vi "Main_Host.vi"() -> ()   [LabVIEW 2020]
doc: "JSMA Project Wizard 0.2.0.11\nRob Humfeld - JET Engineering\nCopyright (c) 2020, JET Engineering"
uses:
  Main_Host_Status STYP.ctl
  <userlib>/JET Engineering/JET_QSM/Code/Private/JET_QSM - Add State [String API].vi
  <userlib>/JET Engineering/JSMA/Libraries/jMasterTable_Message/jMasterTable_Message - Reset.vi
  <userlib>/JET Engineering/JSMA/Libraries/jMasterTable_Module/jMasterTable_Module - Reset.vi
  <userlib>/JET Engineering/JSMA/Libraries/jMasterTable_Message/jMasterTable_Message - Get-Create Queue.vi
  <userlib>/JET Engineering/JSMA/Libraries/jMasterTable_Subscription/jMasterTable_Subscription - Reset.vi
  <userlib>/JET Engineering/JSMA/Libraries/jMasterTable_Module/jMasterTable_Module - Get-Create Queue.vi
  <userlib>/JET Engineering/JSMA/Libraries/jMasterTable_Module/jMasterTable_Module - Get Table Name.vi
  <vilib>/Utility/error.llb/Trim Whitespace.vi
  <userlib>/JET Engineering/JSMA/Libraries/jMasterShutdownFlag/jFlag_MasterShutdown - Reset.vi
  <vilib>/Utility/error.llb/Error Cluster From Error Code.vi
  Shared/Globals/Main_Host Config GBL.vi
  <userlib>/JET Engineering/JSMA/Libraries/jSubscription Class/jSubscription.lvclass
  <userlib>/JET Engineering/JSMA Exception Handler UI/Module_JSMA_UI_ExceptionHandler.lvclass
  <userlib>/JET Engineering/JSMA/Libraries/jApplication/jApplication.lvclass
  Module_UI_TopLevel/Module_UI_TopLevel.lvclass
panel:
  in  "Status":T1
  out "error out":errorcluster
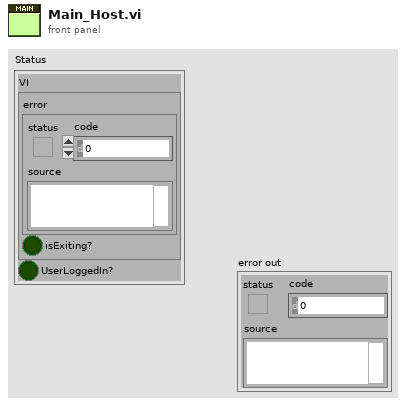
[diagram p1: front panel]
types:
  T1 = typedef "Main_Host_Status STYP.ctl" = cluster{"VI":cluster{"error":errorcluster, "isExiting?":bool}, "UserLoggedIn?":bool}
  T2 = typedef "JET_QSM_Refnum STYP.ctl" = cluster{"state":cluster{"queue":refnum<queue>, "idle":string, "error":string, "STOP":string}, "debug":cluster{"enabled?":bool, "queue":refnum<queue>}, "Invalid.option":T3, "QSM.Name":string}
  T3 = typedef "JET_QSM_InvalidOption STYP.ctl" = enum16{"Ignore", "Dialog", "Error"}
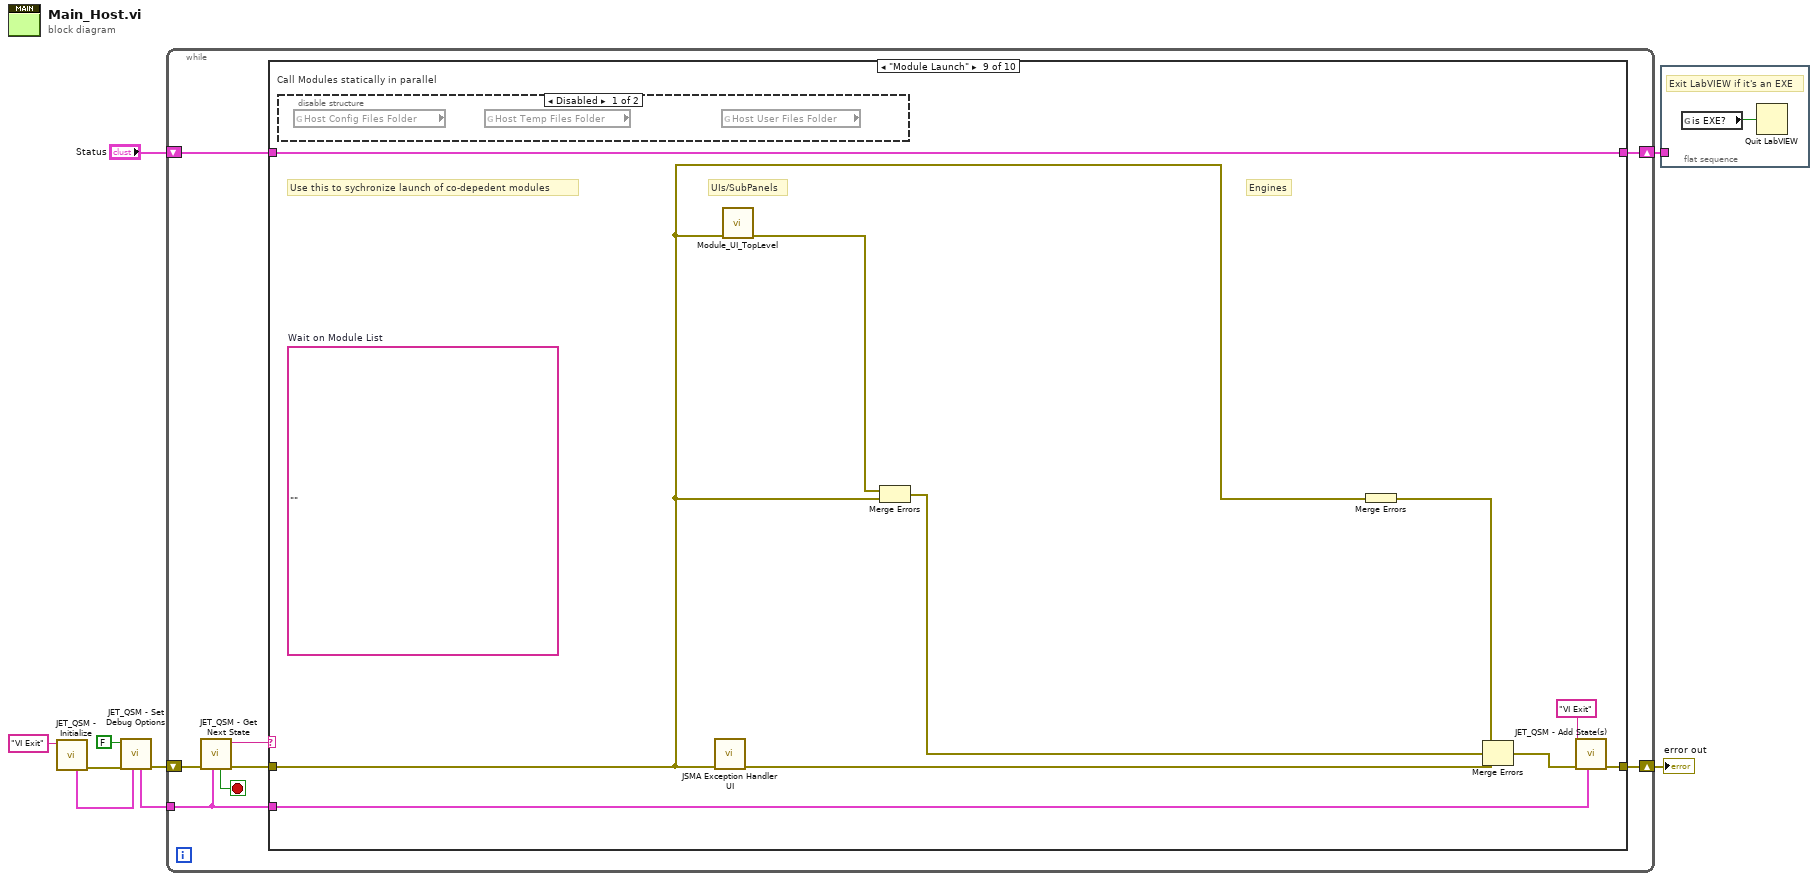
[diagram p0: block diagram]
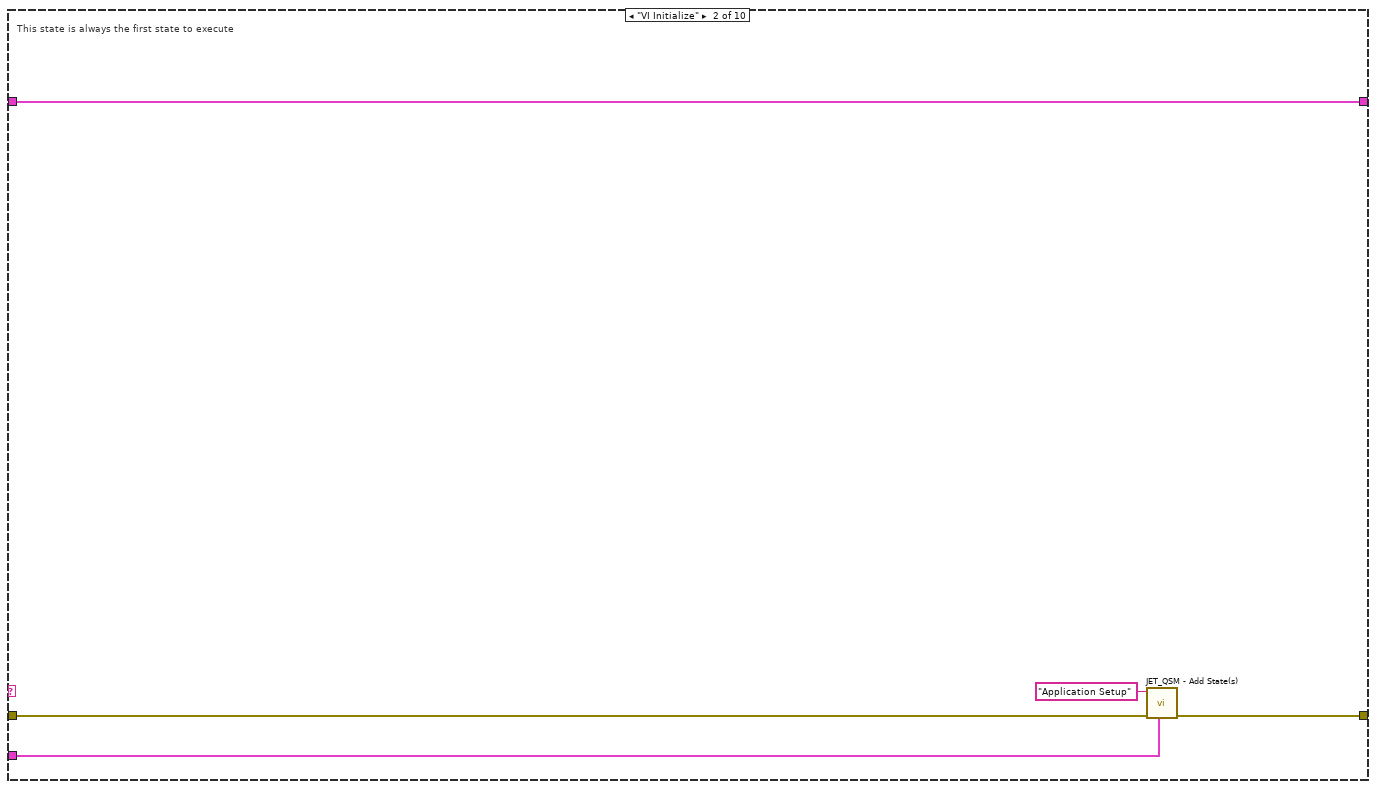
[diagram p3: hidden frame]
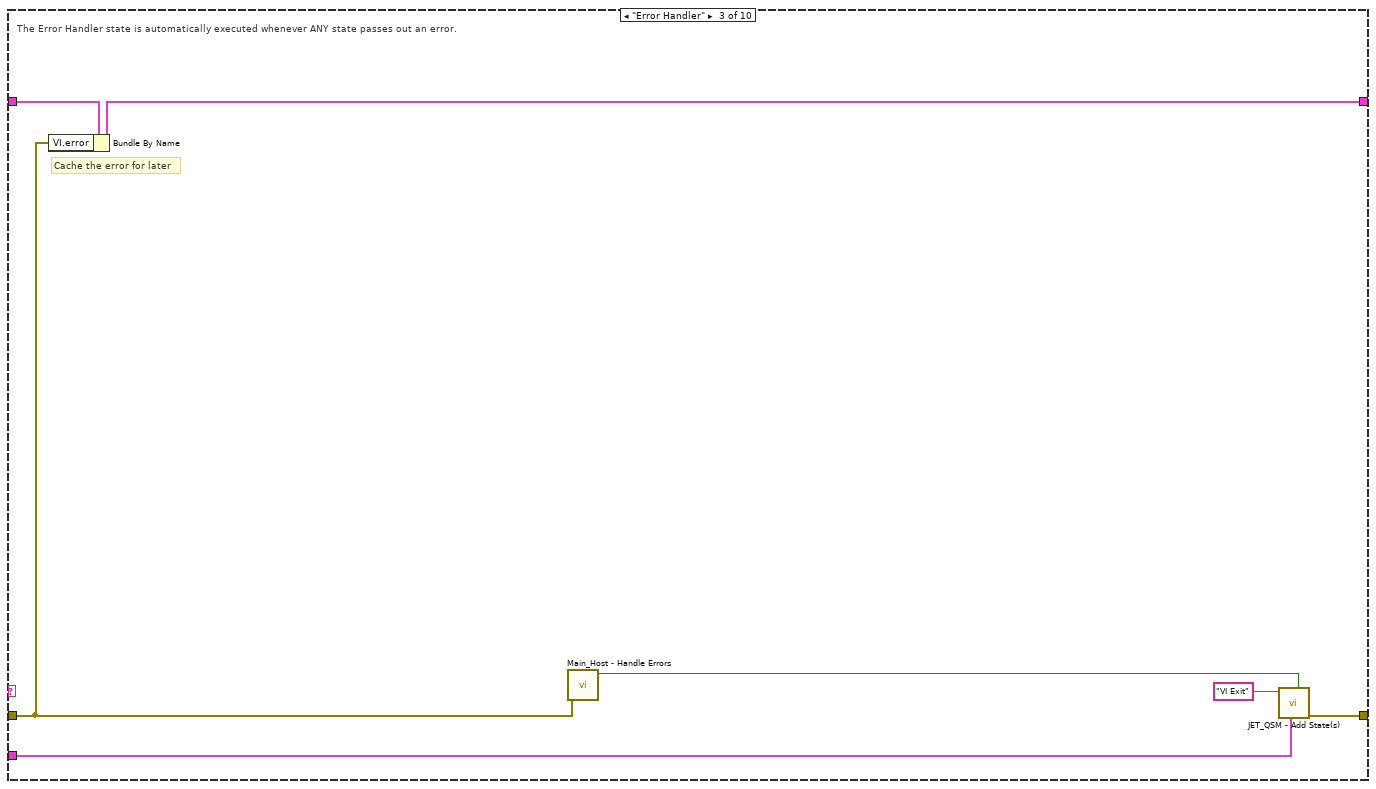
[diagram p4: hidden frame]
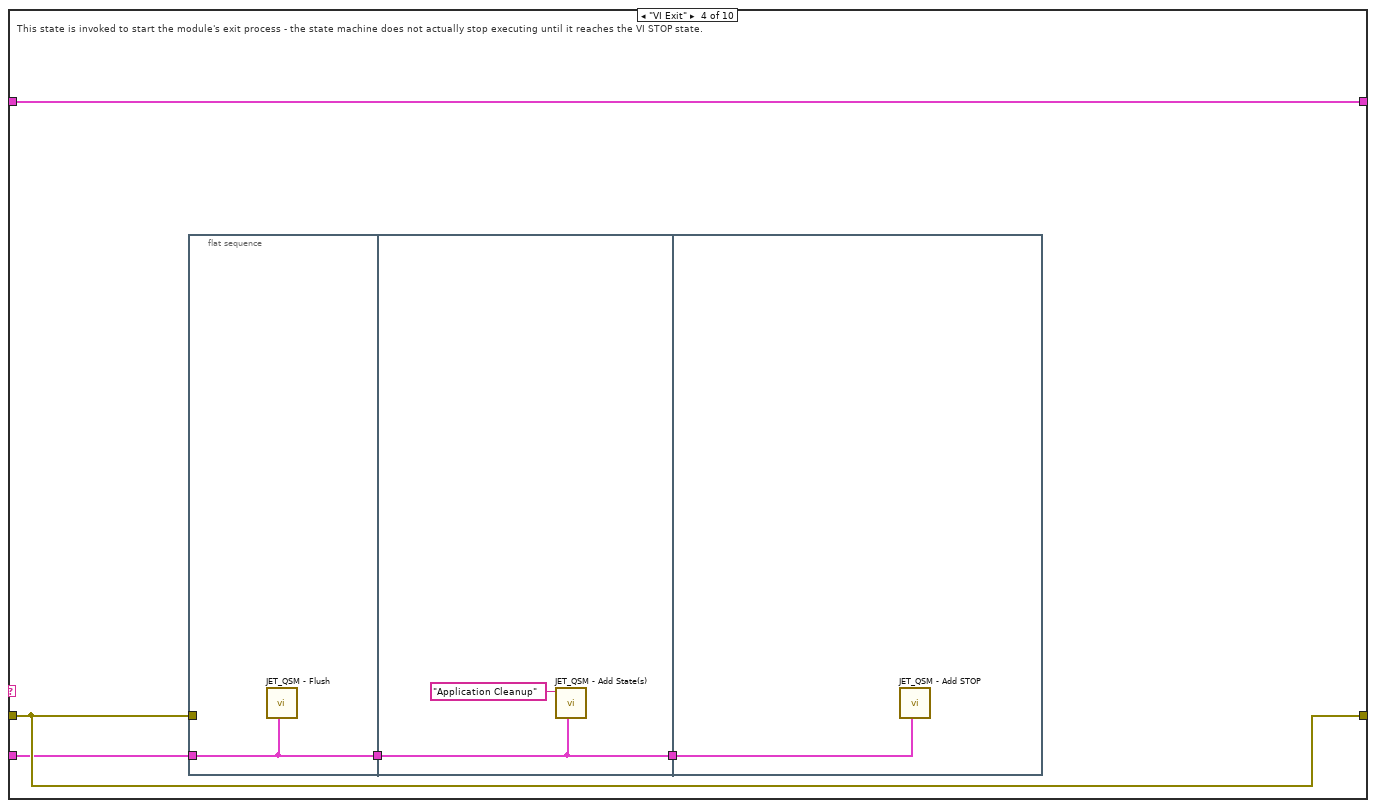
[diagram p5: hidden frame]
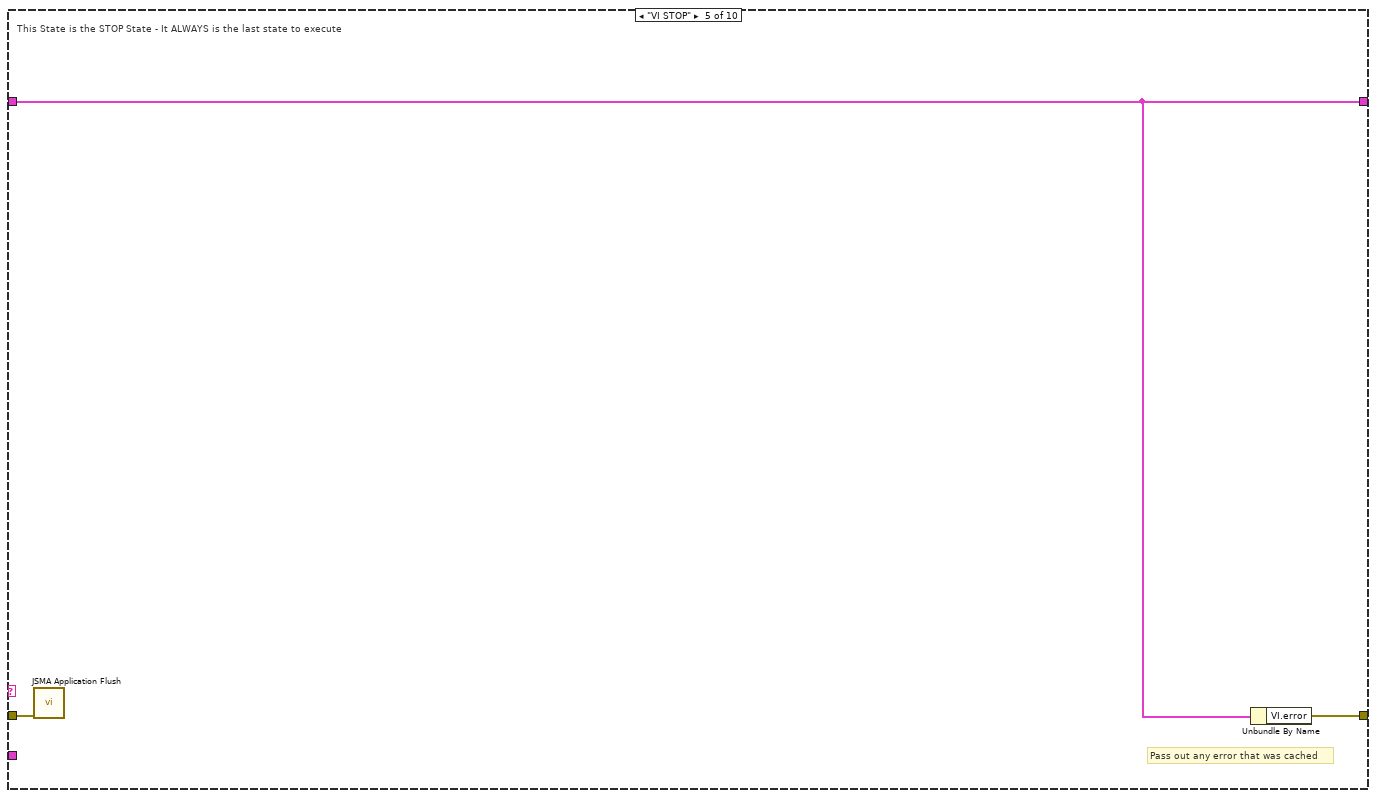
[diagram p6: hidden frame]
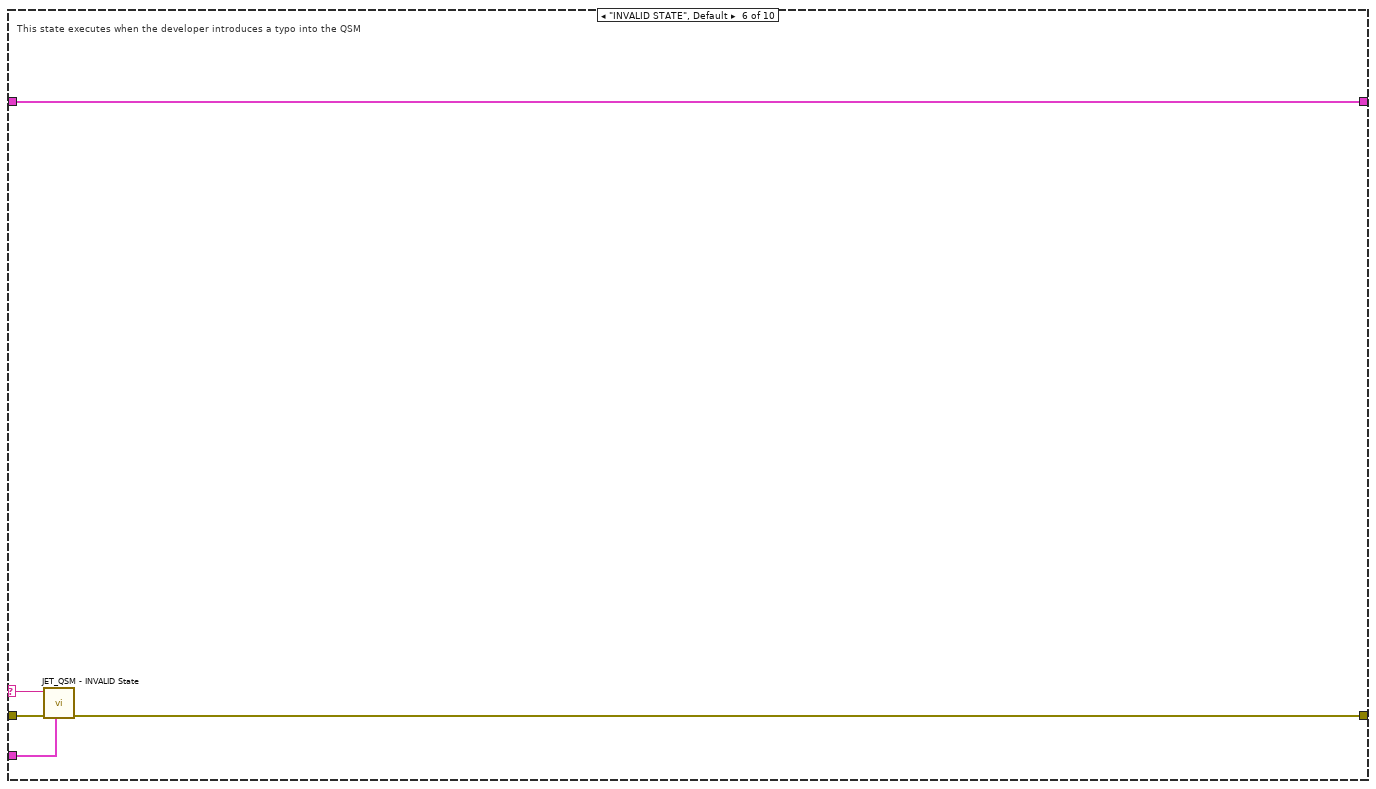
[diagram p7: hidden frame]
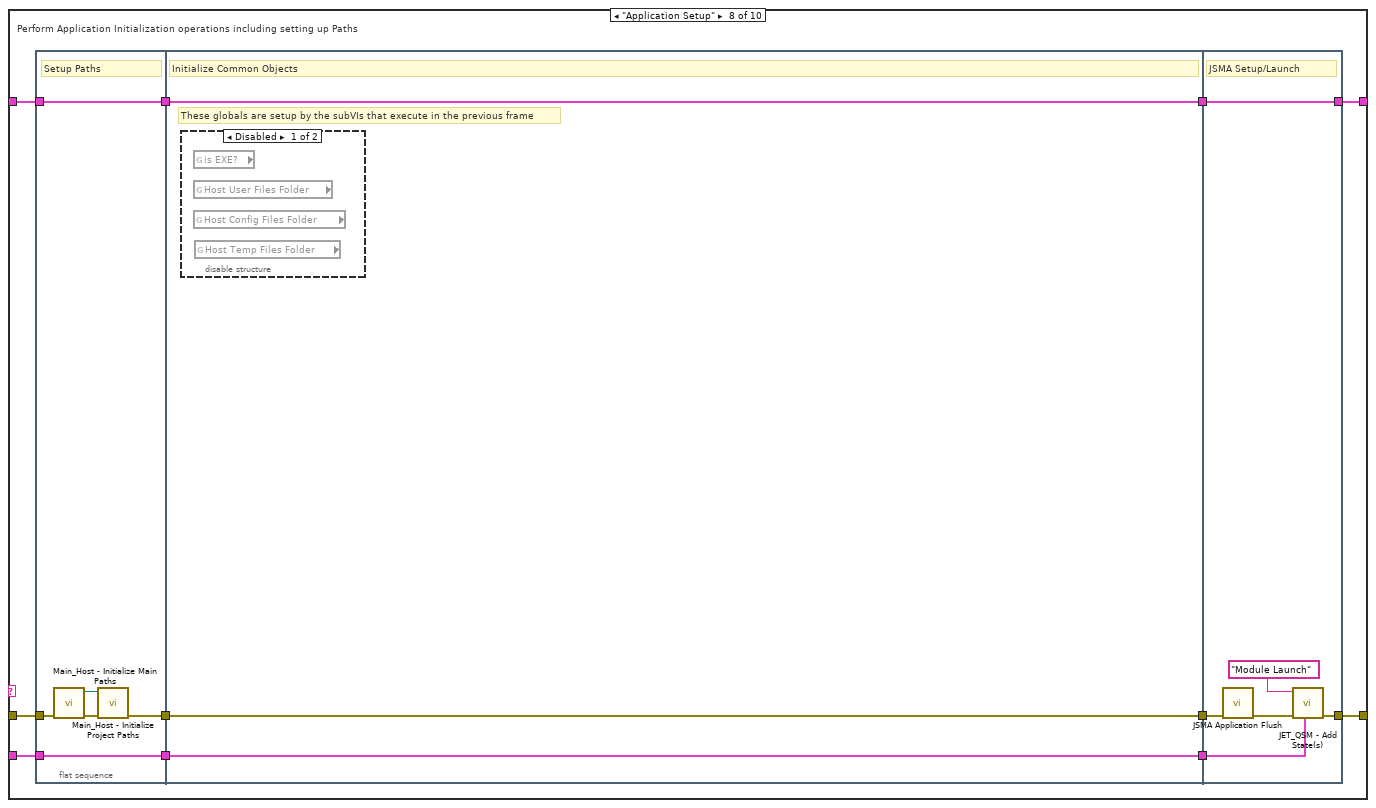
[diagram p9: hidden frame]
diagram:
  n1 = call <userlib>:"JET_QSM - Initialize.vi"("idle state (\"Event Check\")"="VI Exit" ("idle state (\"Event Check\")")) -> ("error out"=w3:errorcluster, "Jet_QSM refnum"=w6:T2)  [unwired: 9 in]
  n2 = call <userlib>:"JET_QSM - Set Debug Options.vi"("Jet_QSM refnum"=w6, "error in (no error)"=w3, "debug.enabled? (F)"=FALSE) -> ("error out"=w4:errorcluster, "Jet_QSM ref"=w5:T2)  [unwired: 7 in]
  n3 = while {
    tunnel: w5 -> [w13]
    shift-right: [w11] -> w2
    shift-left: "Status" -> [w12]
    shift-right: [w10] -> w9
    shift-left: w4 -> [w17]
    stop <- w14 stop-if-true
    n4 = call <userlib>:"JET_QSM - Get Next State.vi"("Jet_QSM refnum"=w13, "error in (no error)"=w17) -> ("error out"=w16:errorcluster, "state"=w15:string, "Stop Loop?"=w14:bool)  [unwired: 5 in, 2 out]
    n5 = case shown="\"Module Launch\"" w15 {
      selector: w15 -> [_ _ _ _ _ w46 _ _ _ _]
      tunnel: w16 -> [w18 w22 w26 w36 w41 w47 w49 w61 w78 w87]
      tunnel: w13 -> [_ w23 w30 w35 _ w45 _ w56 w85 _]
      tunnel: w12 -> [w19 w24 w28 w34 w42 w48 w50 w53 w86 w88]
      tunnel: [w19 w24 w27 w34 w42 w48 w50 w51 w86 w88] -> w11
      tunnel: [w18 w21 w31 w36 w43 w44 w49 w55 w84 w87] -> w10
      frame "------ Standard States ------" {
        # "Standard States are required states for a JET_QSM State Machine\n\nTheir names may be changed; use the Initialize function to specify the new names"
        # "This is a section header; the state is never expected to execute"
      }
      frame "VI Initialize" {
        # "This state is always the first state to execute"
        n6 = call-poly <userlib>:"JET_QSM - Add State(s).vi"("Jet_QSM refnum"=w23, "error in (no error)"=w22, "state(s)"="Application Setup") -> ("error out"=w21:errorcluster)  [unwired: 8 in]
      }
      frame "Error Handler" {
        # "Cache the error for later"
        # "The Error Handler state is automatically executed whenever ANY state passes out an error."
        n7 = Bundle By Name(cluster=w28, "VI.error"=w26) -> (w27:T1)
        n8 = call "Main_Host - Handle Errors.vi"("error in (no error)"=w26) -> ("VI Exit?"=w25:bool)  [unwired: 10 in]
        n9 = call-poly <userlib>:"JET_QSM - Add State(s).vi"("act? (T)"=w25, "Jet_QSM refnum"=w30, "state(s)"="VI Exit") -> ("error out"=w31:errorcluster)  [unwired: 8 in]
      }
      frame "VI Exit" {
        # "This state is invoked to start the module's exit process - the state machine does not actually stop executing until it reaches the VI STOP state."
        n10 = flat-sequence {
          tunnel: w35 -> [w37]
          tunnel: w36 -> [_]
          tunnel: [w37] -> w33
          tunnel: w33 -> [w39]
          tunnel: [w39] -> w32
          tunnel: w32 -> [w40]
          frame #0 {
            n11 = call <userlib>:"JET_QSM - Flush.vi"("Jet_QSM ref"=w37) -> ()  [unwired: 9 in, 2 out]
          }
          frame #1 {
            n12 = call-poly <userlib>:"JET_QSM - Add State(s).vi"("Jet_QSM refnum"=w39, "state(s)"="Application Cleanup") -> ()  [unwired: 9 in, 1 out]
          }
          frame #2 {
            n13 = call <userlib>:"JET_QSM - Add STOP.vi"("Jet_QSM refnum"=w40) -> ()  [unwired: 10 in, 1 out]
          }
        }
      }
      frame "VI STOP" {
        # "Pass out any error that was cached"
        # "This State is the STOP State - It ALWAYS is the last state to execute"
        n14 = call <userlib>:"JSMA Application Flush.vi"("error in (no error)"=w41) -> ()  [unwired: 10 in, 1 out]
        n15 = Unbundle By Name(w42) -> ("VI.error"=w43:errorcluster)
      }
      frame "INVALID STATE", Default {
        # "This state executes when the developer introduces a typo into the QSM"
        n16 = call <userlib>:"JET_QSM - INVALID State.vi"("Jet_QSM refnum"=w45, "error in (no error)"=w47, "state"=w46) -> ("error out"=w44:errorcluster)  [unwired: 8 in]
      }
      frame "------ Actions  ------" {
        # "This is a section header; the state is never expected to execute"
      }
      frame "Application Setup" {
        # "Perform Application Initialization operations including setting up Paths"
        n17 = flat-sequence {
          tunnel: w61 -> [w65]
          tunnel: [w64] -> w60
          tunnel: [w63] -> w57
          tunnel: w56 -> [w63]
          tunnel: [w62] -> w54
          tunnel: w53 -> [w62]
          tunnel: w60 -> [w70]
          tunnel: [w70] -> w59
          tunnel: [w69] -> w58
          tunnel: w57 -> [w69]
          tunnel: w54 -> [w68]
          tunnel: [w68] -> w52
          tunnel: w59 -> [w72]
          tunnel: w58 -> [w74]
          tunnel: [w73] -> w55
          tunnel: w52 -> [w71]
          tunnel: [w71] -> w51
          frame #0 {
            # "Setup Paths"
            n18 = call "Main_Host - Initialize Main Paths.vi"("error in (no error)"=w65) -> ("error out"=w66:errorcluster, "Config Files Folder Path"=w67:path)  [unwired: 8 in, 1 out]
            n19 = call "Main_Host - Initialize Project Paths.vi"("error in (no error)"=w66, "Config Files Folder Path"=w67) -> ("error out"=w64:errorcluster)  [unwired: 8 in, 1 out]
          }
          frame #1 {
            # "These globals are setup by the subVIs that execute in the previous frame"
            # "Initialize Common Objects"
            n20 = disable-structure shown="Disabled" {
              frame Disabled {
                n21 = global read "Main_Host Config GBL.vi" "is EXE?"() -> ()  [unwired: 1 out]
                n22 = global read "Main_Host Config GBL.vi" "Host User Files Folder"() -> ()  [unwired: 1 out]
                n23 = global read "Main_Host Config GBL.vi" "Host Config Files Folder"() -> ()  [unwired: 1 out]
                n24 = global read "Main_Host Config GBL.vi" "Host Temp Files Folder"() -> ()  [unwired: 1 out]
              }
              frame Enabled {
              }
            }
          }
          frame #2 {
            # "JSMA Setup/Launch"
            n25 = call <userlib>:"JSMA Application Flush.vi"("error in (no error)"=w72) -> ("error out"=w76:errorcluster)  [unwired: 10 in]
            n26 = call-poly <userlib>:"JET_QSM - Add State(s).vi"("Jet_QSM refnum"=w74, "error in (no error)"=w76, "state(s)"="Module Launch") -> ("error out"=w73:errorcluster)  [unwired: 8 in]
          }
        }
      }
      frame "Module Launch" {
        (unwired) ""  # Wait on Module List
        # "UIs/SubPanels"
        # "Engines"
        # "Use this to sychronize launch of co-depedent modules"
        # "Call Modules statically in parallel"
        n27 = disable-structure shown="Disabled" {
          frame Disabled {
            n28 = global read "Main_Host Config GBL.vi" "Host Config Files Folder"() -> ()  [unwired: 1 out]
            n29 = global read "Main_Host Config GBL.vi" "Host Temp Files Folder"() -> ()  [unwired: 1 out]
            n30 = global read "Main_Host Config GBL.vi" "Host User Files Folder"() -> ()  [unwired: 1 out]
          }
          frame Enabled {
          }
        }
        n31 = call <userlib>:"JSMA Exception Handler UI.vi"("error in (no error)"=w78) -> ("error out"=w81:errorcluster)  [unwired: 8 in, 2 out]
        n32 = call "Module_UI_TopLevel.vi"("error in (no error)"=w78) -> ("error out"=w77:errorcluster)  [unwired: 10 in]
        n33 = Merge Errors(w77, w78) -> (w80:errorcluster)
        n34 = Merge Errors(w78) -> (w79:errorcluster)
        n35 = Merge Errors(w79, w80, w81) -> (w82:errorcluster)
        n36 = call-poly <userlib>:"JET_QSM - Add State(s).vi"("Jet_QSM refnum"=w85, "error in (no error)"=w82, "state(s)"="VI Exit") -> ("error out"=w84:errorcluster)  [unwired: 8 in]
      }
      frame "Application Cleanup" {
        # "Cleanup Common Objects; This is part of the VI Exiting procedure"
      }
    }
  }
  "error out" <- w9
  n37 = flat-sequence {
    tunnel: w2 -> [_]
    frame #0 {
      # "Exit LabVIEW if it's an EXE"
      n38 = global read "Main_Host Config GBL.vi" "is EXE?"() -> (w89:bool)
      n39 = Quit LabVIEW(quit? (T)=w89) -> ()
    }
  }
